vi "VISA_WRITE.vi"(5 "Value":i32, 7 "Value (str)":string, 8 "error in":errorcluster {"code" format="%.0x"}, 10 "cmd":string, 11 "Session In":refnum<visa-resource-name>="GPIB0::10::INSTR") -> (0 "error out":errorcluster {"code" format="%.0x"}, 3 "Session Out":refnum<visa-resource-name>)   [LabVIEW 2018]
panel:
  out "concatenated string":string
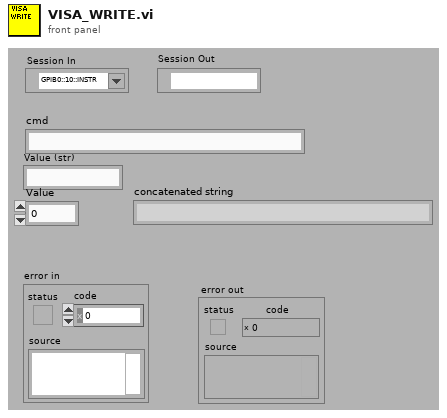
[diagram p1: front panel]
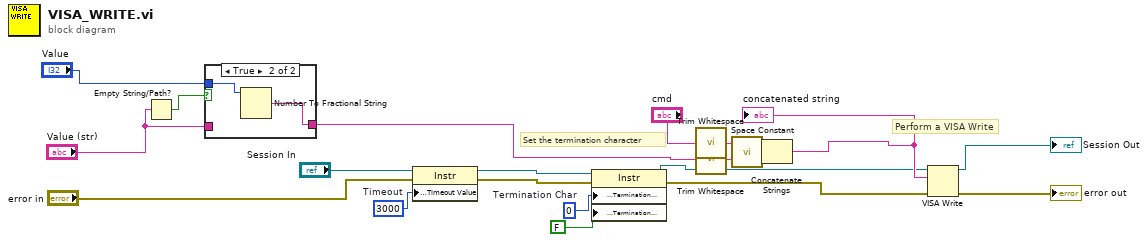
[diagram p0: block diagram]
diagram:
  w15 = u8 0  # Termination Char
  w19 = u32 3000  # Timeout
  # "Perform a VISA Write"
  # "Set the termination character"
  n1 = Empty String/Path?(string/path="Value (str)") -> (empty?=w6:bool)
  n2 = case shown="True" w6 {
    tunnel: "Value (str)" -> [w21 _]
    tunnel: [w21 w23] -> w5
    tunnel: "Value" -> [_ w22]
    frame False {
    }
    frame True {
      n3 = Number To Fractional String(number=w22) -> (F-format string=w23:string)  [unwired: 3 in]
    }
  }
  n4 = property class="Instr"(reference="Session In", error in="error in", "General Settings:Timeout Value"=w19) -> (reference out=w14:refnum<visa-resource-name>, error out=w17:errorcluster)
  n5 = property class="Instr"(reference=w14, error in=w17, "Message Based Settings:Termination Character"=w15, "Message Based Settings:Termination Character Enable"=FALSE ("enable")) -> (reference out=w9:refnum<visa-resource-name>, error out=w16:errorcluster)
  n6 = call <vilib>:"Trim Whitespace.vi"("string"="cmd") -> ("trimmed string"=w3:string)  [unwired: 1 in]
  n7 = call <vilib>:"Trim Whitespace.vi"("string"=w5) -> ("trimmed string"=w2:string)  [unwired: 1 in]
  n8 = call <vilib>:"Space Constant.vi"() -> ("String"=w1:string)
  n9 = Concatenate Strings(w3, w1, w2) -> (w10:string)
  "concatenated string" <- w10
  n10 = VISA Write(VISA resource name=w9, write buffer=w10, error in (no error)=w16) -> (VISA resource name out=→"Session Out":refnum<visa-resource-name>, error out=→"error out":errorcluster)  [unwired: 1 out]
